vi "CompleteTest Saved - Copy.vi"() -> ()   [LabVIEW 2018]
uses:
  <vilib>/myRIO/Common/Instrument Driver Framework/myRIO v1.0/AI/typedefs/AI Channels List.ctl
  <vilib>/myRIO/Common/Instrument Driver Framework/myRIO v1.0/AI/typedefs/AI Channels Enum.ctl
  <vilib>/Studica/Studica Toolkit/Background/PWM Channel.ctl
  <vilib>/Studica/Studica Toolkit/Background/Mxp Selection.ctl
  <vilib>/Studica/Studica Toolkit/Background/I2C Channel.ctl
  <vilib>/Studica/Studica Toolkit/NavX/NavX.lvlib
panel:
  in  "AI Channel":T1=[enum."B/AI1"]
  in  "Position B Servo 3":dbl(slide) scale=-200.0..200.0
  in  "Position B Servo 2":dbl(slide) scale=-200.0..200.0
  in  "Position B Servo 1":dbl(slide) scale=-200.0..200.0
  in  "Position A Servo 3":dbl(slide) scale=-200.0..200.0
  in  "Position A Servo 2":dbl(slide) scale=-200.0..200.0
  in  "Position A Servo 1":dbl(slide) scale=-200.0..200.0
  out "Ping A Inches":fxp<+,64,16>
  out "Ping A cm":fxp<+,64,16>
  out "Ping B Inches":fxp<+,64,16>
  out "Ping B cm":fxp<+,64,16>
  out "Sharp IR Distance":dbl
  out "Distance M1 (inches) B":dbl
  out "Distance M0 (inches) B":dbl
  in  "Reset Encoder 3":bool
  in  "Reset Encoder 2":bool
  in  "Invert M1 B":bool
  in  "Invert M0 B":bool
  in  "Speed M1 B":dbl(slide) scale=-1.0..1.0
  in  "Speed M0 B":dbl(slide) scale=-1.0..1.0
  out "Distance M0 (inches)":dbl
  out "Distance M1 (inches)":dbl
  in  "Reset Encoder 1":bool
  in  "Reset Encoder 0":bool
  in  "Wheel Diameter (inches)":dbl format="%#_13g"
  in  "Ticks Per Rev":u32
  in  "stop":bool
  out "LSB Data":T3
  in  "Thresholds":dbl[](array[numeric])
  in  "Invert M1":bool
  in  "Speed M1":dbl(slide) scale=-1.0..1.0
  in  "Invert M0":bool
  in  "Speed M0":dbl(slide) scale=-1.0..1.0
  out "YRPHfH":T4
  out "Timestamp":u32
  in  "Zero Yaw":bool
  # "Set the encoder ticks \nand wheel diameter here\nfor acurate distance"
  # "Motors will only stop when \na value of 0 is applied"
  # "MXP B"
  # "MXP A"
  # "Press here to Zero the yaw"
  # "If stop is hit, motors will stop\nand robot will have to be reset\nbefore normal operation can \ncontinue."
  # "Set the LSB\nthresholds here\na value in the middle \nis best. Range (0-5)"
  # "MXP A\nPWM 3"
  # "MXP A\nPWM 4"
  # "MXP B\nPWM 3"
  # "MXP A\nPWM 2"
  # "MXP B\nPWM 2"
  # "MXP B\nPWM 3"
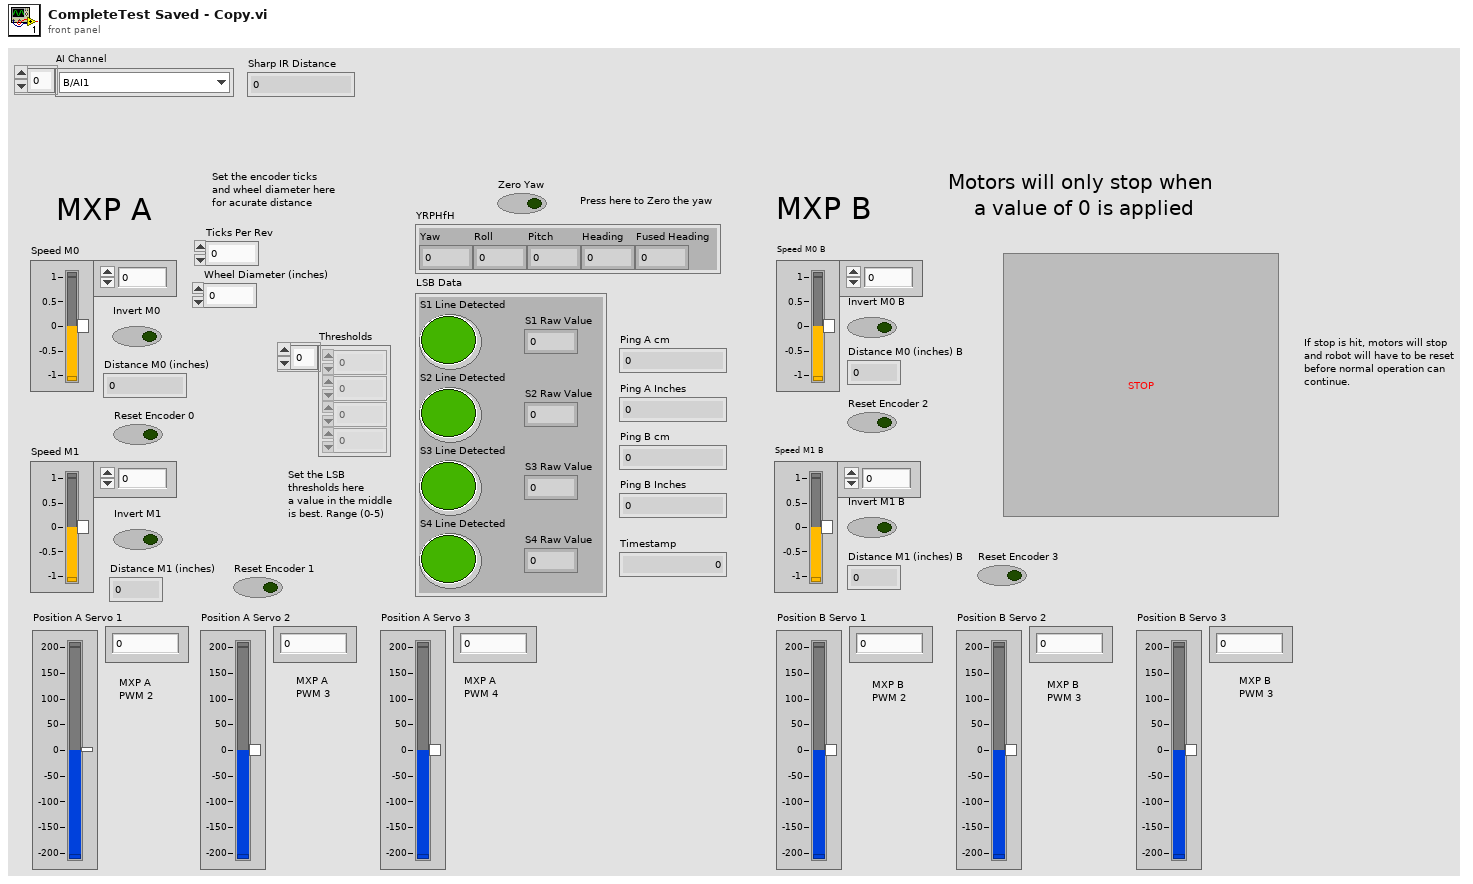
[diagram p1: front panel]
types:
  T1 = typedef "AI Channels List.ctl" = T2[]
  T2 = typedef "AI Channels Enum.ctl" = enum16{"Not Connected", "AudioIn/Left", "AudioIn/Right", "C/AI0", "C/AI1", "A/AI0", "A/AI1", "A/AI2", "A/AI3", "A/AI4", "A/AI5", "A/AI6", "A/AI7", "B/AI0", "B/AI1", "B/AI2", "B/AI3", "B/AI4", "B/AI5", "B/AI6", "B/AI7", "AI/AI0", "AI/AI1", "AI/AI2", "AI/AI3", "A/AI0 (DIFF)", "A/AI1 (DIFF)", "A/AI2 (DIFF)", "A/AI3 (DIFF)", "B/AI0 (DIFF)", "B/AI1 (DIFF)", "B/AI2 (DIFF)", "B/AI3 (DIFF)"}
  T3 = cluster{"S1 Line Detected":bool, "S2 Line Detected":bool, "S3 Line Detected":bool, "S4 Line Detected":bool, "S1 Raw Value":dbl, "S2 Raw Value":dbl, "S3 Raw Value":dbl, "S4 Raw Value":dbl}
  T4 = cluster{"Yaw":dbl, "Roll":dbl, "Pitch":dbl, "Heading":dbl, "Fused Heading":dbl}
  T5 = typedef "PWM Channel.ctl" = enum16{"Not Connected", "A/PWM0", "A/PWM1", "A/PWM2", "A/PWM3", "A/PWM4", "B/PWM0", "B/PWM1", "B/PWM2", "B/PWM3", "B/PWM4", "C/PWM0", "C/PWM1"}
  T6 = typedef "Mxp Selection.ctl" = enum16{"MXP A", "MXP B"}
  T7 = typedef "I2C Channel.ctl" = enum16{"Not Connected", "A", "B"}
  T8 = cluster{"I2C Ref Out":cluster{"I2C Channel":T7, "FPGA VI Reference Out":refnum<k20>}, "Connected":bool, "Slave Address (7-bit)":u8, "Registry":u8[]}
  T9 = cluster{"PWM Channel":T5, "FPGA VI Reference Out":refnum<k20>}
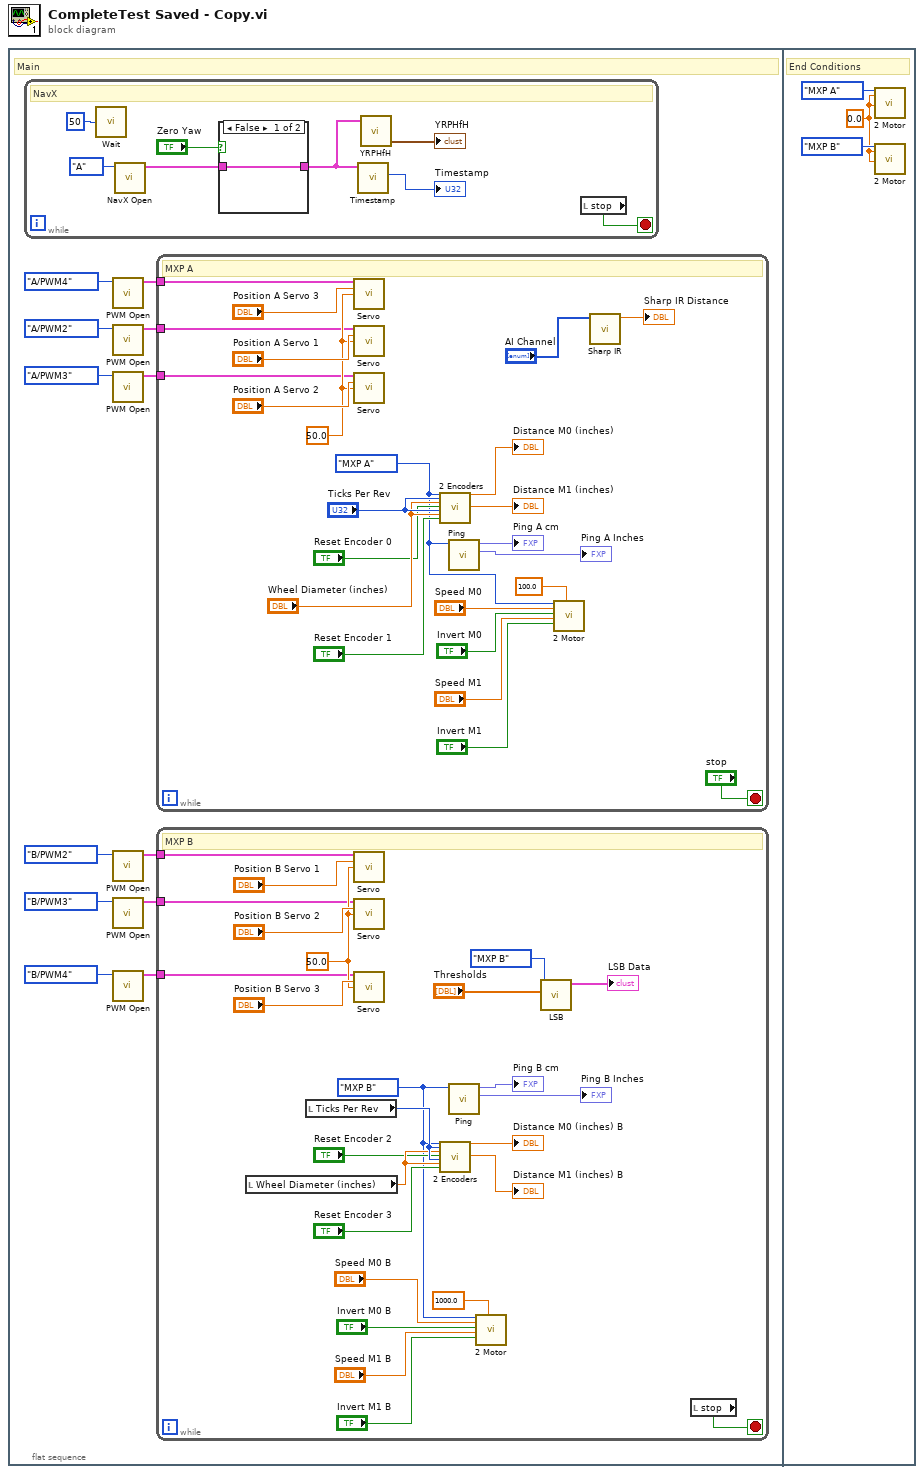
[diagram p0: block diagram]
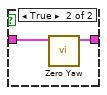
[diagram p2: hidden frame]
diagram:
  n1 = flat-sequence {
    frame #0 {
      # "Main"
      n2 = while {
        stop <- w38 stop-if-true
        # "NavX"
        n3 = call "Wait"("Count(mSec)"=u32 50) -> ()  [unwired: 1 out]
        n4 = call <vilib>:"NavX Open.vi"("I2C Channel"=I2C_Channel."A") -> ("NavX Info"=w42:T8)  [unwired: 9 in, 1 out]
        n5 = case shown="False" "Zero Yaw" {
          tunnel: w42 -> [w46 w48]
          tunnel: [w46 w47] -> w43
          frame False {
          }
          frame True {
            n6 = call <vilib>:"Zero Yaw.vi"("NavX Info In"=w48) -> ("NavX Info Out"=w47:T8)  [unwired: 10 in]
          }
        }
        n7 = call <vilib>:"Timestamp.vi"("NavX Info In"=w43) -> ("Timestamp"=→"Timestamp":u32)  [unwired: 9 in, 1 out]
        n8 = call <vilib>:"YRPHfH.vi"("NavX Info In"=w43) -> ("YRPHfH"=→"YRPHfH":T4)  [unwired: 3 in, 1 out]
        n9 = local read "stop"() -> (w38:bool)
      }
      n10 = call <vilib>:"PWM Open.vi"("PWM Channel"=PWM_Channel."A/PWM4") -> ("PWM Info Out"=w9:T9)  [unwired: 9 in, 1 out]
      n11 = call <vilib>:"PWM Open.vi"("PWM Channel"=PWM_Channel."A/PWM2") -> ("PWM Info Out"=w7:T9)  [unwired: 9 in, 1 out]
      n12 = call <vilib>:"PWM Open.vi"("PWM Channel"=PWM_Channel."A/PWM3") -> ("PWM Info Out"=w8:T9)  [unwired: 9 in, 1 out]
      n13 = call <vilib>:"PWM Open.vi"("PWM Channel"=PWM_Channel."B/PWM2") -> ("PWM Info Out"=w3:T9)  [unwired: 9 in, 1 out]
      n14 = call <vilib>:"PWM Open.vi"("PWM Channel"=PWM_Channel."B/PWM3") -> ("PWM Info Out"=w2:T9)  [unwired: 9 in, 1 out]
      n15 = call <vilib>:"PWM Open.vi"("PWM Channel"=PWM_Channel."B/PWM4") -> ("PWM Info Out"=w1:T9)  [unwired: 9 in, 1 out]
      n16 = while {
        tunnel: w9 -> [w54]
        tunnel: w8 -> [w53]
        tunnel: w7 -> [w52]
        stop <- "stop" stop-if-true
        w55 = 50.0
        w61 = Mxp_Selection."MXP A" ("Mxp Side")
        # "MXP A"
        n17 = call <vilib>:"Servo.vi"("PWM Info In"=w54, "Position"="Position A Servo 3", "Frequency [Hz]"=w55) -> ()  [unwired: 11 in, 2 out]
        n18 = call <vilib>:"Servo.vi"("PWM Info In"=w52, "Position"="Position A Servo 1", "Frequency [Hz]"=w55) -> ()  [unwired: 11 in, 2 out]
        n19 = call <vilib>:"Servo.vi"("PWM Info In"=w53, "Position"="Position A Servo 2", "Frequency [Hz]"=w55) -> ()  [unwired: 11 in, 2 out]
        n20 = call <vilib>:"2 Encoders.vi"("Mxp Side"=w61, "Ticks Per Rev M0"="Ticks Per Rev", "Wheel Diameter M0 (inches)"="Wheel Diameter (inches)", "Reset Encoder 0"="Reset Encoder 0", "Ticks Per Rev M1"="Ticks Per Rev", "Wheel Diameter M1 (inches)"="Wheel Diameter (inches)", "Reset Encoder 1"="Reset Encoder 1") -> ("Distance M0 (inches)"=→"Distance M0 (inches)":dbl, "Distance M1 (inches)"=→"Distance M1 (inches)":dbl)  [unwired: 18 in, 1 out]
        n21 = call <vilib>:"Ping.vi"("Mxp Side"=w61) -> ("IN"=→"Ping A Inches":fxp<+,64,16>, "CM"=→"Ping A cm":fxp<+,64,16>)  [unwired: 8 in, 1 out]
        n22 = call <vilib>:"2 Motor.vi"("Mxp Side"=w61, "Speed M0"="Speed M0", "Invert M0"="Invert M0", "Speed M1"="Speed M1", "Invert M1"="Invert M1", "Frequency [Hz]"=100.0) -> ()  [unwired: 13 in, 1 out]
        n23 = call <vilib>:"Sharp IR.vi"("AI Channel"="AI Channel") -> ("Sharp IR Distance"=→"Sharp IR Distance":dbl)  [unwired: 8 in, 2 out]
      }
      n24 = while {
        tunnel: w3 -> [w18]
        tunnel: w2 -> [w17]
        tunnel: w1 -> [w16]
        stop <- w37 stop-if-true
        w19 = 50.0
        w25 = Mxp_Selection."MXP B" ("Mxp Side")
        # "MXP B"
        n25 = local read "Wheel Diameter (inches)"() -> (w30:dbl)
        n26 = local read "Ticks Per Rev"() -> (w31:u32)
        n27 = call <vilib>:"Servo.vi"("PWM Info In"=w18, "Position"="Position B Servo 1", "Frequency [Hz]"=w19) -> ()  [unwired: 11 in, 2 out]
        n28 = call <vilib>:"Servo.vi"("PWM Info In"=w17, "Position"="Position B Servo 2", "Frequency [Hz]"=w19) -> ()  [unwired: 11 in, 2 out]
        n29 = call <vilib>:"Servo.vi"("PWM Info In"=w16, "Position"="Position B Servo 3", "Frequency [Hz]"=w19) -> ()  [unwired: 11 in, 2 out]
        n30 = call <vilib>:"2 Encoders.vi"("Mxp Side"=w25, "Ticks Per Rev M0"=w31, "Wheel Diameter M0 (inches)"=w30, "Reset Encoder 0"="Reset Encoder 2", "Ticks Per Rev M1"=w31, "Wheel Diameter M1 (inches)"=w30, "Reset Encoder 1"="Reset Encoder 3") -> ("Distance M0 (inches)"=→"Distance M0 (inches) B":dbl, "Distance M1 (inches)"=→"Distance M1 (inches) B":dbl)  [unwired: 18 in, 1 out]
        n31 = call <vilib>:"Ping.vi"("Mxp Side"=w25) -> ("IN"=→"Ping B Inches":fxp<+,64,16>, "CM"=→"Ping B cm":fxp<+,64,16>)  [unwired: 8 in, 1 out]
        n32 = call <vilib>:"2 Motor.vi"("Mxp Side"=w25, "Speed M0"="Speed M0 B", "Invert M0"="Invert M0 B", "Speed M1"="Speed M1 B", "Invert M1"="Invert M1 B", "Frequency [Hz]"=1000.0) -> ()  [unwired: 13 in, 1 out]
        n33 = call <vilib>:"LSB.vi"("Thresholds"="Thresholds", "Mxp Side"=Mxp_Selection."MXP B") -> ("LSB Data"=→"LSB Data":T3)  [unwired: 8 in, 1 out]
        n34 = local read "stop"() -> (w37:bool)
      }
    }
    frame #1 {
      w73 = 0.0
      # "End Conditions"
      n35 = call <vilib>:"2 Motor.vi"("Mxp Side"=Mxp_Selection."MXP A", "Speed M0"=w73, "Speed M1"=w73) -> ()  [unwired: 16 in, 1 out]
      n36 = call <vilib>:"2 Motor.vi"("Mxp Side"=Mxp_Selection."MXP B", "Speed M0"=w73, "Speed M1"=w73) -> ()  [unwired: 16 in, 1 out]
    }
  }
